vi "SoftwareNote.vi"() -> ()   [LabVIEW 2020]
panel:
  in  "Stop":bool
  out "Avaiable function":string
  out "String":string
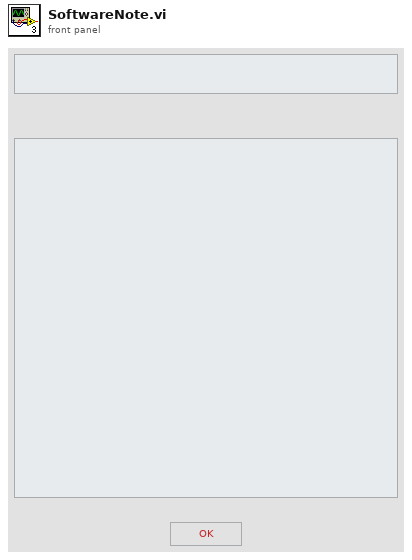
[diagram p1: front panel]
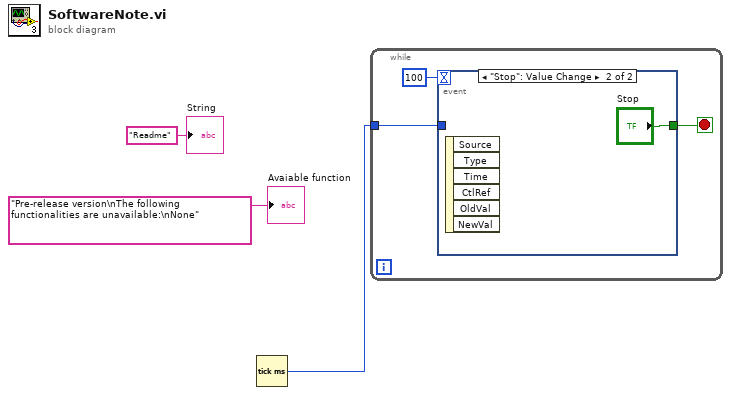
[diagram p0: block diagram]
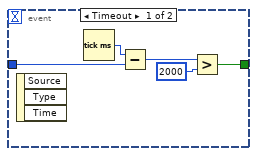
[diagram p2: hidden frame]
diagram:
  n1 = Tick Count (ms)() -> (millisecond timer value=w1:u32)
  n2 = while {
    tunnel: w1 -> [w5]
    stop <- w6 stop-if-true
    n3 = event shown="[1] \"Stop\": Value Change" {
      selector: _ -> [_ _]
      dyn-events: _ -> [_ _]
      timeout: 100 -> [_ _]
      tunnel: [w7 "Stop"] -> w6
      tunnel: w5 -> [w10 _]
      event Timeout {
        n4 = event-data() -> ()  [unwired: 1 in, 3 out]
        n5 = Tick Count (ms)() -> (millisecond timer value=w11:u32)
        n6 = Subtract(x=w11, y=w10) -> (x-y=w9:u32)
        n7 = Greater?(x=w9, y=u32 2000) -> (0:w7:bool)
      }
      event "Stop": Value Change {
        n8 = event-data() -> ()  [unwired: 1 in, 6 out]
      }
    }
  }
  "String" <- "Readme" ("String")
  "Avaiable function" <- "Pre-release version\nThe following functionalities are unavailable:\nNone" ("String")
